vi "Close.vi"(8 "Error In":errorcluster, 11 "CS++MessageLogger in":refnum<class "CS++MessageLogger.lvclass">) -> (0 "Error Out":errorcluster, 3 "CS++MessageLogger out":refnum<class "CS++MessageLogger.lvclass">)   [LabVIEW 2014, in "CS++BaseClasses.lvlib" / "CS++MessageLogger.lvclass"]
doc: "Close the message logger."
uses:
  CS++MessageLogger.lvclass
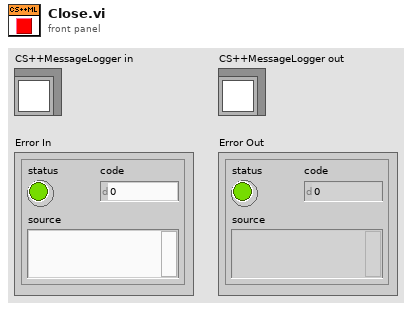
[diagram p1: front panel]
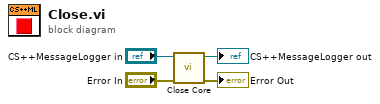
[diagram p0: block diagram]
diagram:
  n1 = call-dynamic "Close Core.vi"("Error In"="Error In", "CS++MessageLogger in"="CS++MessageLogger in") -> ("Error Out"=→"Error Out":errorcluster, "CS++MessageLogger out"=→"CS++MessageLogger out":refnum<class "CS++MessageLogger.lvclass">)  [unwired: 8 in]
